vi "Create Set Coin Output String.vi"(0 "Cell Index":i32, 5 "Zero Indexed? (T)":bool=TRUE, 11 "error in (no error)":errorcluster) -> (4 "Output Text":string, 15 "error out":errorcluster)   [LabVIEW 2014]
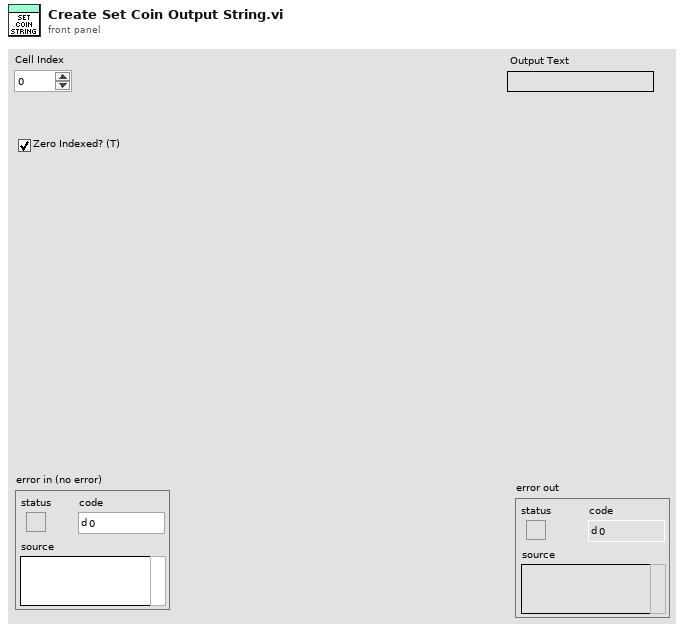
[diagram p1: front panel]
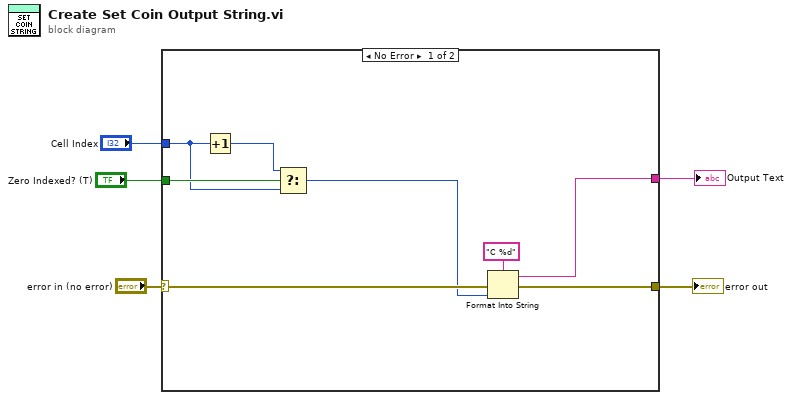
[diagram p0: block diagram]
diagram:
  n1 = case shown="No Error" "error in (no error)" {
    selector: "error in (no error)" -> [w12 w14]
    tunnel: [w11 w14] -> w4
    tunnel: "Cell Index" -> [w7 _]
    tunnel: [w10 _] -> w2
    tunnel: "Zero Indexed? (T)" -> [w9 _]
    frame No Error {
      n2 = Increment(x=w7) -> (x+1=w8:i32)
      n3 = Select(t=w8, s=w9, f=w7) -> (s? t:f=w6:i32)
      n4 = Format Into String(format string="C %d", error in=w12, w6) -> (resulting string=w10:string, error out=w11:errorcluster)  [unwired: 1 in]
    }
    frame Error {
    }
  }
  "error out" <- w4
  "Output Text" <- w2
